vi "Motic Set RGB Gain Value.vi"(0 "camera":i32, 5 "r":sgl, 7 "g":sgl, 9 "b":sgl, 11 "error in (no error)":errorcluster) -> (4 "camera out":i32, 6 "ri out":i32, 8 "bi out":i32, 10 "gi out":i32, 15 "error out":errorcluster)   [LabVIEW 2012, in "MoticApi.lvlib"]
doc: "MOTICAPI bool Motic_SetRGBGainValue(MUCam_Handle camera, float r, float g, float b, int *ri, int *gi, int *bi);"
uses:
  MoticApi.lvlib
  MoticApi.dll
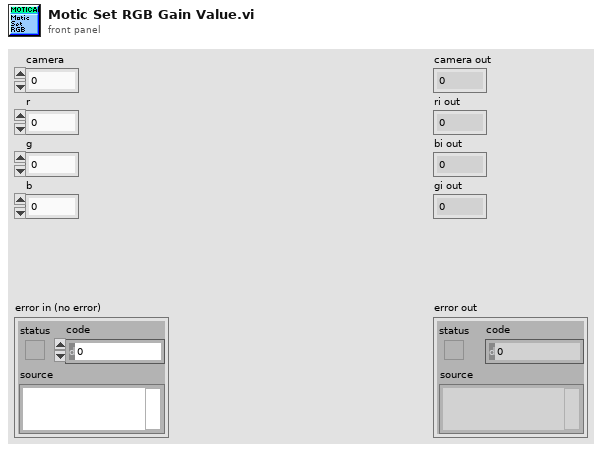
[diagram p1: front panel]
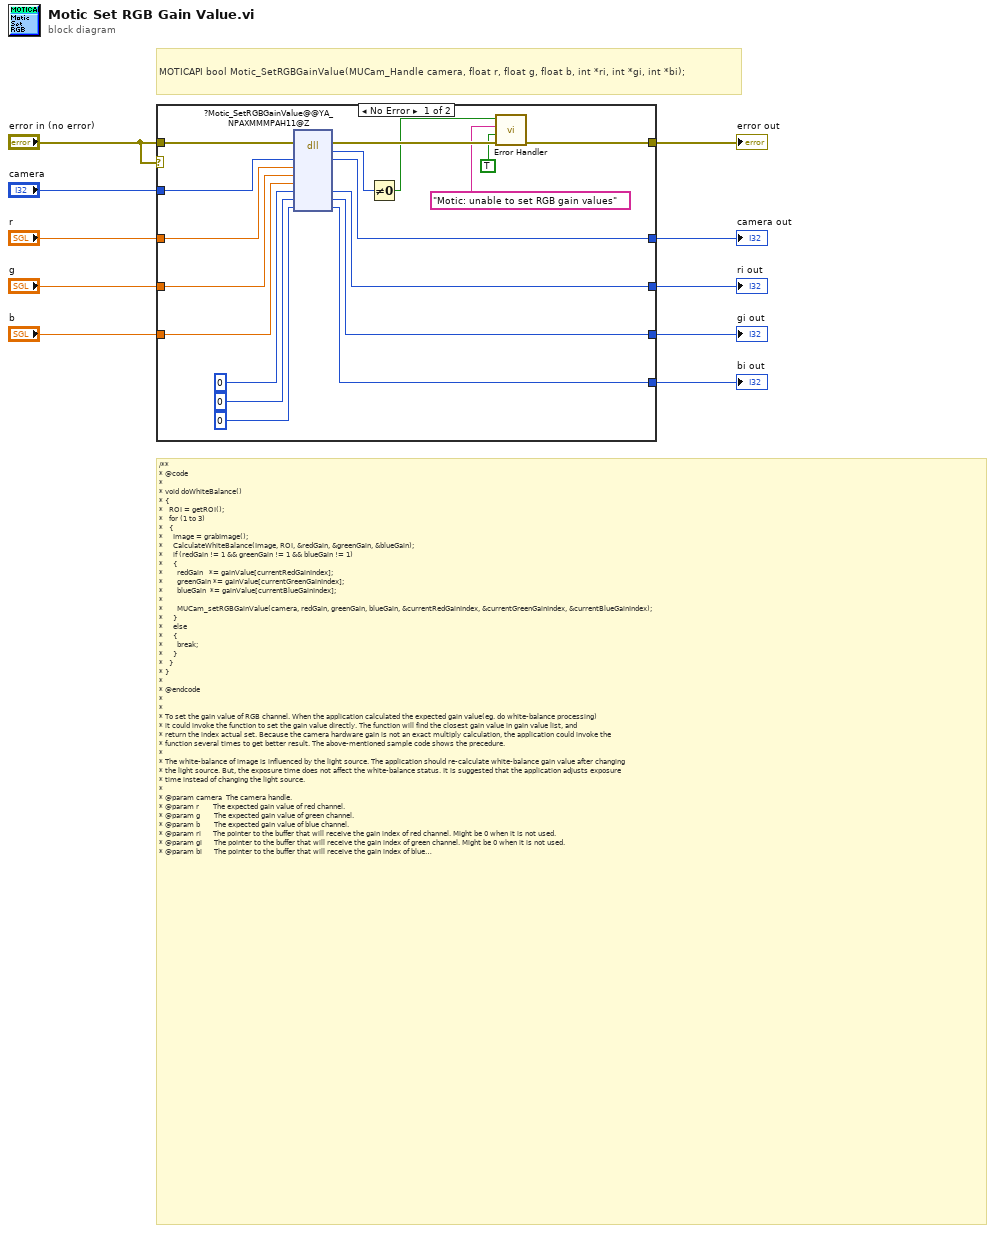
[diagram p0: block diagram]
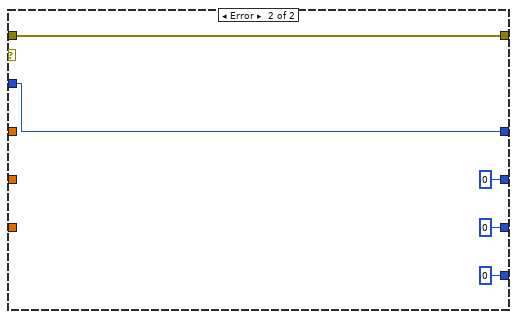
[diagram p2: hidden frame]
diagram:
  # "/**\n* @code\n*\n* void doWhiteBalance()\n* {\n*   ROI = getROI();\n*   for (1 to 3)\n*   {\n*     Image = grabImage();\n*     CalculateWhiteBalance(Image, ROI, &redGain, &greenGain, &blueGain);\n*     if (redGain != 1 && greenGain != 1 && blueGain != 1)\n*     {\n*       redGain   *= gainValue[currentRedGainIndex];\n*       greenGain *= gainValue[currentGreenGainIndex];\n*       blueGain  *= gainValue[currentBlueGainIndex];\n*\n*       MUCam_setRGBGainValue(camera, redGain, greenGain, blueGain, &currentRedGainIndex, &currentGreenGainIndex, &currentBlueGainIndex);\n*     }\n*     else\n*     {\n*       break;\n*     }\n*   }\n* }\n*\n* @endcode\n*\n*\n* To set the gain value of RGB channel. When the application calculated the expected gain value(eg. do white-balance processing)\n* it could invoke the function to set the gain value directly. The function will find the closest gain value in gain value list, and\n* return the index actual set. Because the camera hardware gain is not an exact multiply calculation, the application could invoke the\n* function several times to get better result. The above-mentioned sample code shows the precedure.\n*\n* The white-balance of image is influenced by the light source. The application should re-calculate white-balance gain value after changing\n* the light source. But, the exposure time does not affect the white-balance status. It is suggested that the application adjusts exposure\n* time instead of changing the light source.\n*\n* @param camera  The camera handle.\n* @param r       The expected gain value of red channel.\n* @param g       The expected gain value of green channel.\n* @param b       The expected gain value of blue channel.\n* @param ri      The pointer to the buffer that will receive the gain index of red channel. Might be 0 when it is not used.\n* @param gi      The pointer to the buffer that will receive the gain index of green channel. Might be 0 when it is not used.\n* @param bi      The pointer to the buffer that will receive the gain index of blue channel. Might be 0 when it is not used.\n*\n* @return        True if successful; False if failed.\n*\n* @attention     Some camears don't support different gain values in RGB channels. The function will return true only when the parameters r,g,b are the same.\n*\n* @see MUCam_getGainCount, MUCam_setRGBGainIndex\n*/"
  # "MOTICAPI bool Motic_SetRGBGainValue(MUCam_Handle camera, float r, float g, float b, int *ri, int *gi, int *bi);"
  n1 = case shown="No Error" "error in (no error)" {
    tunnel: "camera" -> [w27 w32]
    tunnel: [w26 w32] -> w9
    tunnel: "r" -> [w25 _]
    tunnel: "g" -> [w24 _]
    tunnel: "b" -> [w23 _]
    tunnel: [w22 0 ("ri")] -> w5
    tunnel: [w21 0 ("gi")] -> w4
    tunnel: [w20 0 ("bi")] -> w3
    tunnel: "error in (no error)" -> [w19 w33]
    tunnel: [w18 w33] -> w2
    frame No Error {
      n2 = dll-call lib="C:/Users/TTS-Digital/Desktop/MoticApi/MoticApi_git/MoticApi/MoticApi.*" fn="?Motic_SetRGBGainValue@@YA_NPAXMMMPAH11@Z"(error in=w19, "camera"=w27, "r"=w25, "g"=w24, "b"=w23, "ri"=0, "gi"=0, "bi"=0) -> (error out=w17:errorcluster, "return type"=w28:u8, "camera"=w26:i32, "ri"=w22:i32, "gi"=w21:i32, "bi"=w20:i32)  [unwired: 5 in, 1 out]
      n3 = Not Equal To 0?(x=w28) -> (x != 0?=w16:bool)
      n4 = call "Error Handler.vi"("error in (no error)"=w17, "Is warning?"=TRUE, "Error message"="Motic: unable to set RGB gain values", "Function return"=w16) -> ("error out"=w18:errorcluster)  [unwired: 7 in]
    }
    frame Error {
    }
  }
  "camera out" <- w9
  "ri out" <- w5
  "gi out" <- w4
  "bi out" <- w3
  "error out" <- w2
